vi "Test.vi"() -> ()   [LabVIEW 2019]
uses:
  <vilib>/vision/Image Controls.llb/IMAQ Image.ctl
panel:
  in  "Bool":bool
  out "Image":T1(plugin-control)
  out "OutCluster":T2
  out "ErrorOut":errorcluster
  in  "stop":bool
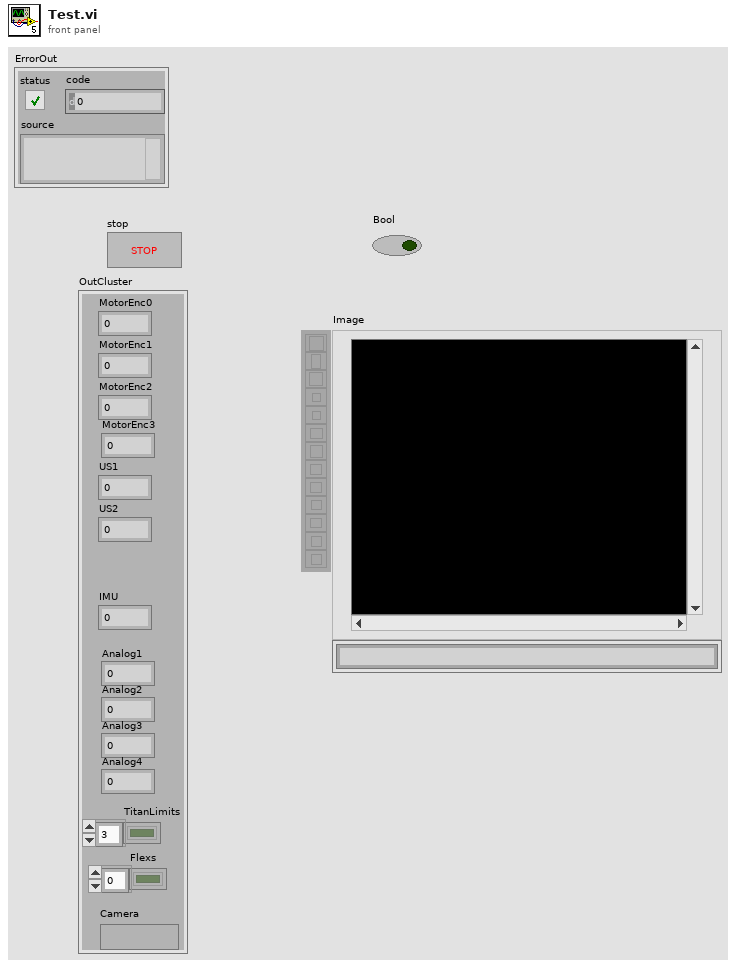
[diagram p1: front panel]
types:
  T1 = typedef "IMAQ Image.ctl" = refnum<image>
  T2 = cluster{"MotorEnc0":dbl, "MotorEnc1":dbl, "MotorEnc2":dbl, "MotorEnc3":dbl, "US1":dbl, "US2":dbl, "Analog1":dbl, "Analog2":dbl, "Analog3":dbl, "Analog4":dbl, "IMU":dbl, "TitanLimits":bool[], "Flexs":bool[], "Camera":T1}
  T3 = cluster{"ListenData":refnum<k24>, "ListenCamera":refnum<k24>, "TalkData":refnum<k24>}
  T4 = cluster{"MotorSpeed0":dbl, "MotorSpeed1":dbl, "MotorSpeed2":dbl, "MotorSpeed3":dbl, "HCDIO 1":dbl, "HCDIO 2":dbl, "HCDIO 3":dbl, "HCDIO 4":dbl, "HCDIO 5":dbl, "HCDIO 6":dbl, "HCDIO 7":dbl, "HCDIO 8":dbl, "HCDIO 9":dbl, "HCDIO 10":dbl}
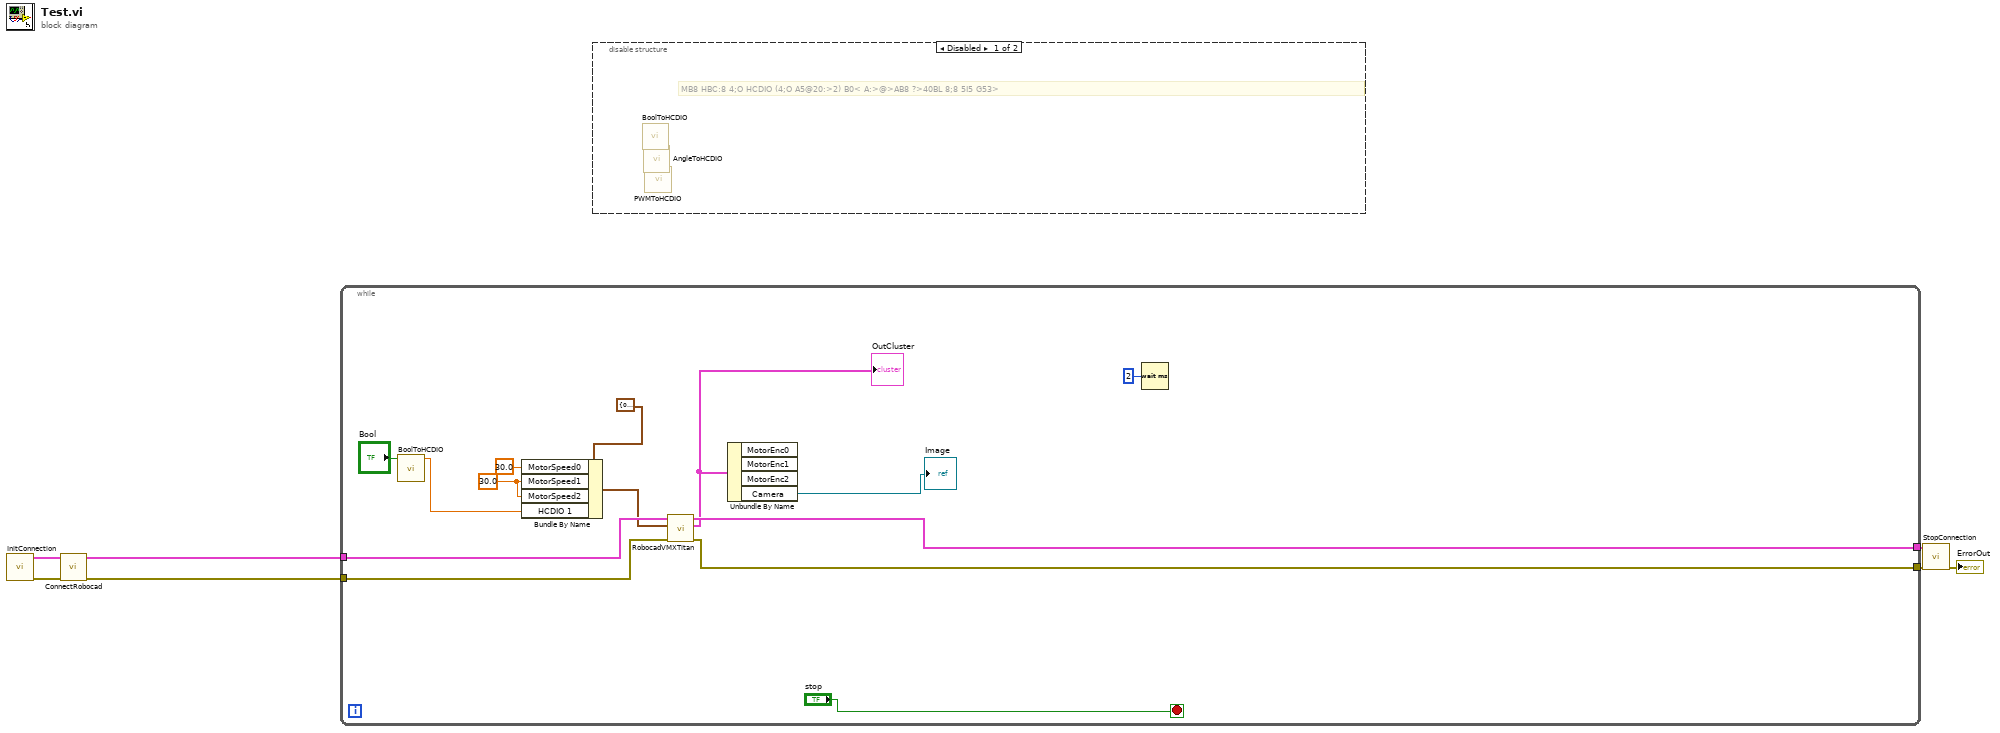
[diagram p0: block diagram]
diagram:
  n1 = call "InitConnection.vi"() -> ("ErrorOut"=w5:errorcluster, "OutConnection"=w6:T3)  [unwired: 10 in]
  n2 = call "ConnectRobocad.vi"("ErrorIn"=w5, "Reference"=w6) -> ("ErrorOut"=w3:errorcluster, "OutConnection"=w4:T3)  [unwired: 8 in]
  n3 = while {
    tunnel: w4 -> [w17]
    tunnel: w3 -> [w20]
    tunnel: [w19] -> w2
    tunnel: [w18] -> w1
    stop <- "stop" stop-if-true
    w11 = 30.0 ("MotorSpeed1")
    n4 = call "BoolToHCDIO.vi"("Bool"="Bool") -> ("Out"=w9:dbl)  [unwired: 10 in]
    n5 = Bundle By Name(cluster=T4 {"MotorSpeed0"=0.0, "MotorSpeed1"=0.0, "MotorSpeed2"=0.0, "MotorSpeed3"=0.0, "HCDIO 1"=0.0, "HCDIO 2"=0.0, "HCDIO 3"=0.0, "HCDIO 4"=0.0, "HCDIO 5"=0.0, "HCDIO 6"=0.0, "HCDIO 7"=0.0, "HCDIO 8"=0.0, "HCDIO 9"=0.0, "HCDIO 10"=0.0} ("InCluster"), "MotorSpeed0"=30.0, "MotorSpeed1"=w11, "MotorSpeed2"=w11, "HCDIO 1"=w9) -> (w15:T4)
    n6 = call "RobocadVMXTitan.vi"("ErrorIn"=w20, "InCluster"=w15, "Reference"=w17) -> ("ErrorOut"=w19:errorcluster, "OutCluster"=w16:T2, "OutReference"=w18:T3)  [unwired: 6 in]
    "OutCluster" <- w16
    n7 = Unbundle By Name(w16) -> ("Camera"=→"Image":T1)  [unwired: 3 out]
    n8 = Wait (ms)(milliseconds to wait=u32 2) -> ()  [unwired: 1 out]
  }
  n9 = disable-structure shown="Disabled" {
    frame Disabled {
      # "MB8 HBC:8 4;O HCDIO (4;O A5@20:>2) B0< A:>@>AB8 ?>40BL 8;8 5I5 G53>"
      n10 = call "BoolToHCDIO.vi"() -> ()  [unwired: 11 in, 1 out]
      n11 = call "AngleToHCDIO.vi"() -> ()  [unwired: 11 in, 1 out]
      n12 = call "PWMToHCDIO.vi"() -> ()  [unwired: 11 in, 1 out]
    }
    frame Enabled {
    }
  }
  n13 = call "StopConnection.vi"("ErrorIn"=w2, "Reference"=w1) -> ("ErrorOut"=→"ErrorOut":errorcluster)  [unwired: 9 in]
